vi "database.vi"(6 "Age":string, 7 "Nationality":string, 9 "Surname":string, 10 "Name":string, 11 "Action":T1) -> (3 "sorted 2D array":string[][](array[string]))   [LabVIEW 2023]
uses:
  3f864bc0-539d-4c5e-9c10-e3e9bc990849.vi
  #typedef_action.ctl
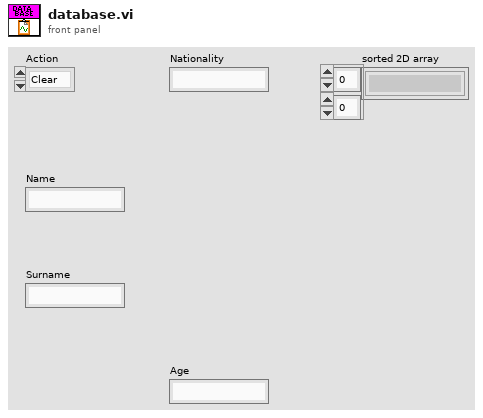
[diagram p1: front panel]
types:
  T1 = typedef "#typedef_action.ctl" = enum16{"Clear", "Add", "Sort"}
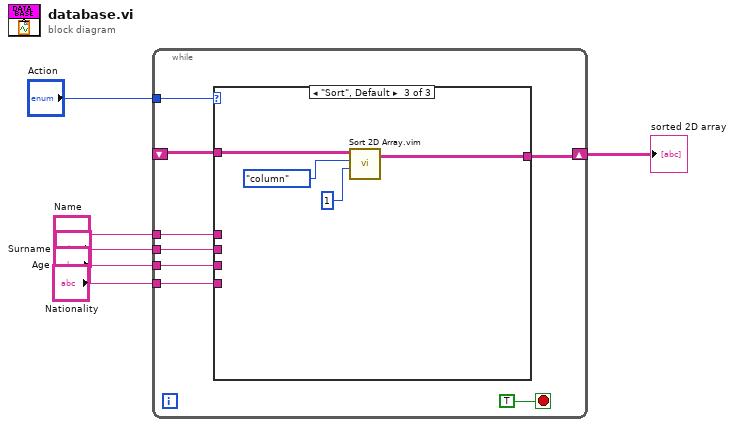
[diagram p0: block diagram]
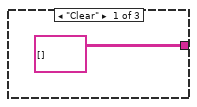
[diagram p2: hidden frame]
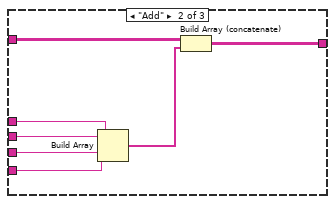
[diagram p3: hidden frame]
diagram:
  n1 = while {
    shift-right: [w7] -> w6
    shift-left: _ -> [w8]
    tunnel: "Action" -> [w13]
    tunnel: "Name" -> [w12]
    tunnel: "Surname" -> [w11]
    tunnel: "Age" -> [w10]
    tunnel: "Nationality" -> [w9]
    stop <- TRUE stop-if-true
    n2 = case shown="\"Sort\", Default" w13 {
      tunnel: w12 -> [_ w22 _]
      tunnel: w11 -> [_ w21 _]
      tunnel: w10 -> [_ w20 _]
      tunnel: w9 -> [_ w19 _]
      tunnel: w8 -> [_ w17 w26]
      tunnel: [string[][] [] w16 w25] -> w7
      frame "Clear" {
      }
      frame "Add" {
        n3 = Build Array(w22, w21, w20, w19) -> (w18:string[])
        n4 = Build Array (concatenate)(w17, w18) -> (w16:string[][])
      }
      frame "Sort", Default {
        n5 = call "Sort 2D Array.vim"("index"=1, "dimension to index (column)"=enum16{"column", "row"}."column", "2D array"=w26) -> ("sorted 2D array"=w25:string[][])  [unwired: 7 in, 1 out]
      }
    }
  }
  "sorted 2D array" <- w6
